vi "Test Compare Inequal Enums.vi"(8 "error in (no error)":errorcluster, 11 "Compare Assertion Test In":refnum<class "Compare Assertion Test.lvclass">) -> (0 "error out":errorcluster, 3 "Compare Assertion Test Out":refnum<class "Compare Assertion Test.lvclass">)   [LabVIEW 2020, in "LUnit Tests.lvlib" / "Compare Assertion Test.lvclass"]
uses:
  Compare Assertion Test.lvclass
  Compare Assertion Test.lvclass/Compare Assertion Test.ctl
  Test Dummys/Test Case Test Double/Test Case Test Double.lvclass
  <vilib>/Astemes/LUnit/Test Case.lvclass
  source/Framework/Result Classes/Assertion Result/Public/TypeDefs/Status.ctl
  source/Framework/Result Classes/Assertion Result/Assertion Result.lvclass
  C:/Program Files (x86)/National Instruments/LabVIEW 2020/vi.lib/Astemes/LUnit/Test Case.lvclass
  C:/Users/anton/Documents/GitHub/LUnit/tests/Compare Assertion Test/Compare Assertion Test.lvclass
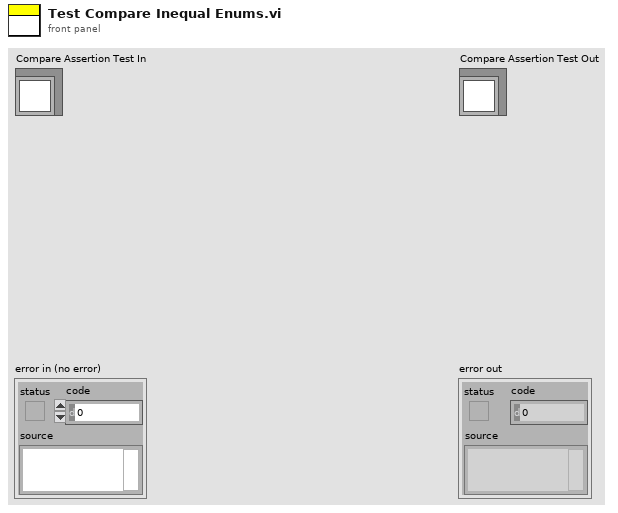
[diagram p1: front panel]
types:
  T1 = typedef "Assertion Result.lvclass/Status.ctl" = enum16{"Pass", "Fail", "Error", "Skipped", "Setup Error", "Broken", "Teardown Error"}
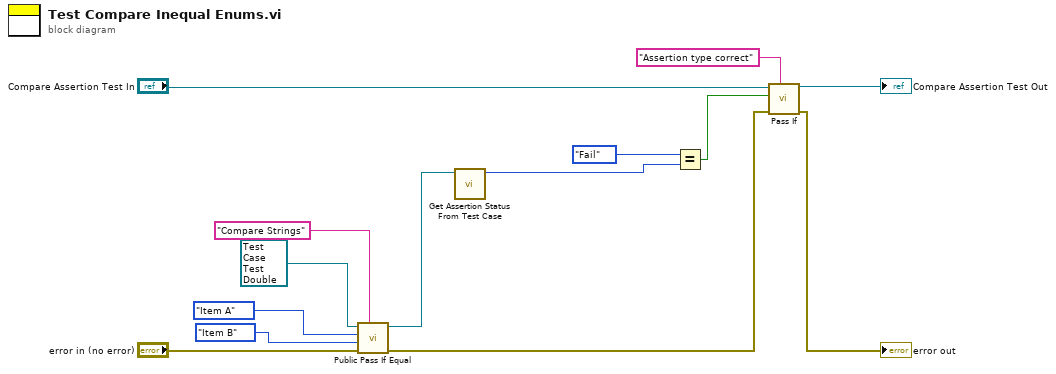
[diagram p0: block diagram]
diagram:
  n1 = call "Public Pass If Equal.vi"("Description"="Compare Strings", "error in (no error)"="error in (no error)", "Actual"=enum16{"Item A", "Item B"}."Item B", "Expected"=enum16{"Item A", "Item B"}."Item A", "Test Case Test Double in"=refnum<class "Test Case Test Double.lvclass"> refnum ("Test Case Test Double.lvclass")) -> ("error out"=w10:errorcluster, "Test Case Test Double out"=w9:refnum<class "Test Case Test Double.lvclass">)  [unwired: 5 in]
  n2 = call "Get Assertion Status From Test Case.vi"("Test Case Test Double in"=w9) -> ("Status"=w8:T1)  [unwired: 10 in]
  n3 = Equal?(x=Status."Fail", y=w8) -> (x = y?=w13:bool)
  n4 = call <vilib>:"Pass If.vi"("Description"="Assertion type correct", "error in (no error)"=w10, "Pass?"=w13, "LUnit Test Case In"="Compare Assertion Test In") -> ("error out"=→"error out":errorcluster, "LUnit Test Case Out"=→"Compare Assertion Test Out":refnum<class "Compare Assertion Test.lvclass">)  [unwired: 6 in]
